vi "Square Pulse Options String.vi"(8 "Error In":errorcluster, 11 "Square Pulse Options":T1 {"Threshold %" min=0.0 max=100.0}) -> (0 "Error Out":errorcluster, 3 "Option String":string)   [LabVIEW 2021, in "Fits.lvlib"]
uses:
  Square Pulse Options.ctl
  Square Pulse Levels Type.ctl
  Fits.lvlib
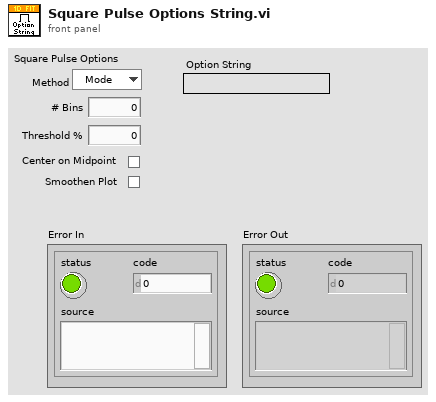
[diagram p1: front panel]
types:
  T1 = typedef "Fits.lvlib/Square Pulse Options.ctl" = cluster{"Method":T2, "# Bins":i32, "Threshold %":dbl, "Center on Midpoint":bool, "Smoothen Plot":bool}
  T2 = typedef "Fits.lvlib/Square Pulse Levels Type.ctl" = enum16{"Mode", "Mean"}
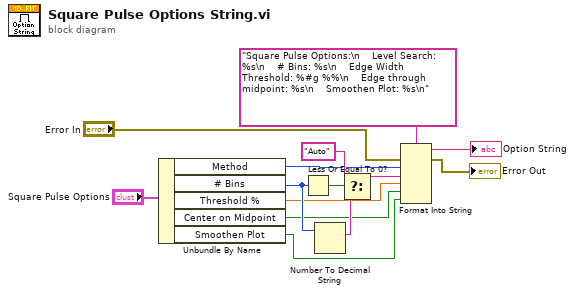
[diagram p0: block diagram]
diagram:
  n1 = Unbundle By Name("Square Pulse Options") -> ("Method"=w5:T2, "# Bins"=w13:i32, "Threshold %"=w6:dbl, "Center on Midpoint"=w7:bool, "Smoothen Plot"=w1:bool)
  n2 = Less Or Equal To 0?(x=w13) -> (x <= 0?=w10:bool)
  n3 = Number To Decimal String(number=w13) -> (decimal integer string=w14:string)  [unwired: 1 in]
  n4 = Select(t="Auto" ("input 2"), s=w10, f=w14) -> (s? t:f=w12:string)
  n5 = Format Into String(format string="Square Pulse Options:\n    Level Search: %s\n    # Bins: %s\n    Edge Width Threshold: %#g %%\n    Edge through midpoint: %s\n    Smoothen Plot: %s\n", error in="Error In", w5, w12, w6, w7, w1) -> (resulting string=→"Option String":string, error out=→"Error Out":errorcluster)  [unwired: 1 in]
